vi "shag_start — 9.vi"() -> ()   [LabVIEW 2016]
uses:
  <vilib>/Instr/_visa.llb/VISA Configure Serial Port (Instr).vi
panel:
  out "положение в мин 4":i32
  out "text4":string
  out "4":i32
  out "3":i32
  out "положение в мин 3":i32
  out "text3":string
  out "text":string
  out "2":i32
  out "1":i32
  out "text2":string
  out "положение в мин 2":i32
  out "положение в мин 1":i32
  in  "all":T1(tab)
  out "положение шд 2":i32(knob) scale=-10.0..190.0
  out "текущее положение 2":string
  out "положение в минутах 2":string
  in  "Минуты 2":i32 min=-600 max=11400
  in  "Stop двигатель 2":bool
  in  "Вращение по градусам +  2":bool
  in  "Вращение по градусам -  2":bool
  in  "Вернуться в нулевое положение 2":bool
  in  "Задать текущее положение нулевым 2":bool
  in  "Установка минут 2":bool
  in  "Блокировать трубку №2":bool
  out "положение шд":i32(knob) scale=-10.0..190.0
  out "текущее положение":string
  out "положение в минутах 1":string
  in  "Минуты":i32 min=-600 max=11400
  in  "Stop двигатель":bool
  in  "Вращение по градусам +":bool
  in  "Вращение по градусам -":bool
  in  "Вернуться в нулевое положение":bool
  in  "Задать текущее положение нулевым":bool
  in  "Установка минут":bool
  in  "Блокировать зеркало №1":bool
  in  "stop":bool
  out "положение шд 3":i32(knob) scale=-10.0..190.0
  out "текущее положение 3":string
  out "положение в минутах 3":string
  in  "Минуты 3":i32 min=-600 max=11400
  in  "Stop двигатель 3":bool
  in  "Вращение по градусам +  3":bool
  in  "Вращение по градусам -  3":bool
  in  "Вернуться в нулевое положение 3":bool
  in  "Задать текущее положение нулевым 3":bool
  in  "Установка минут 3":bool
  in  "Блокировать стол №3":bool caption="Блокировать трубку №2"
  out "положение шд 4":i32(knob) scale=-10.0..190.0
  out "текущее положение 4":string
  out "положение в минутах 4":string
  in  "Минуты 4":i32 min=-600 max=11400
  in  "Stop двигатель 4":bool
  in  "Вращение по градусам +  4":bool
  in  "Вращение по градусам -  4":bool
  in  "Вернуться в нулевое положение 4":bool
  in  "Задать текущее положение нулевым 4":bool
  in  "Установка минут 4":bool
  in  "Блокировать стол №3 2":bool caption="Блокировать трубку №2"
  in  "Выберете COM порт":refnum<visa-resource-name>="COM1"
  in  "Скорость обмена данными":u32(ring)=19200 items=["9600"=9600, "19200"=19200, "38400"=38400, "57600"=57600]
  in  "Число бит на символ":u16=8 min=5 max=8 step=1
  in  "Контроль чётности":enum16{"None", "Odd", "Even", "Mark", "Space"}(ring)
  in  "Стоповый бит":u16(ring)=10 items=["1.0"=10, "1.5"=15, "2.0"=20]
  in  "Контроль переполнения":u16(ring) items=["None"=0, "XON/XOFF"=1, "RTS/CTS"=2, "DTR/DSR"=4]
  # "1 - адресс 1 двигателя\n2 - адресс 2 двигателя\n$0MV\\01+   - запуск всех двигателей в положительном направлении \n$0MS\\00   - остановка всех двигателей\n$0MJ\\04+\\00\\00\\01   - 1 шаг всех двигателей\n$0SS\\01\\10   - скорость 10 для всех двигателей"
  # "Ренгеновская трубка №2"
  # "Положение:"
  # "Зеркало №1"
  # "Положение:"
  # "Поворотный стол №3"
  # "Положение:"
  # "Счётчик №4"
  # "Положение:"
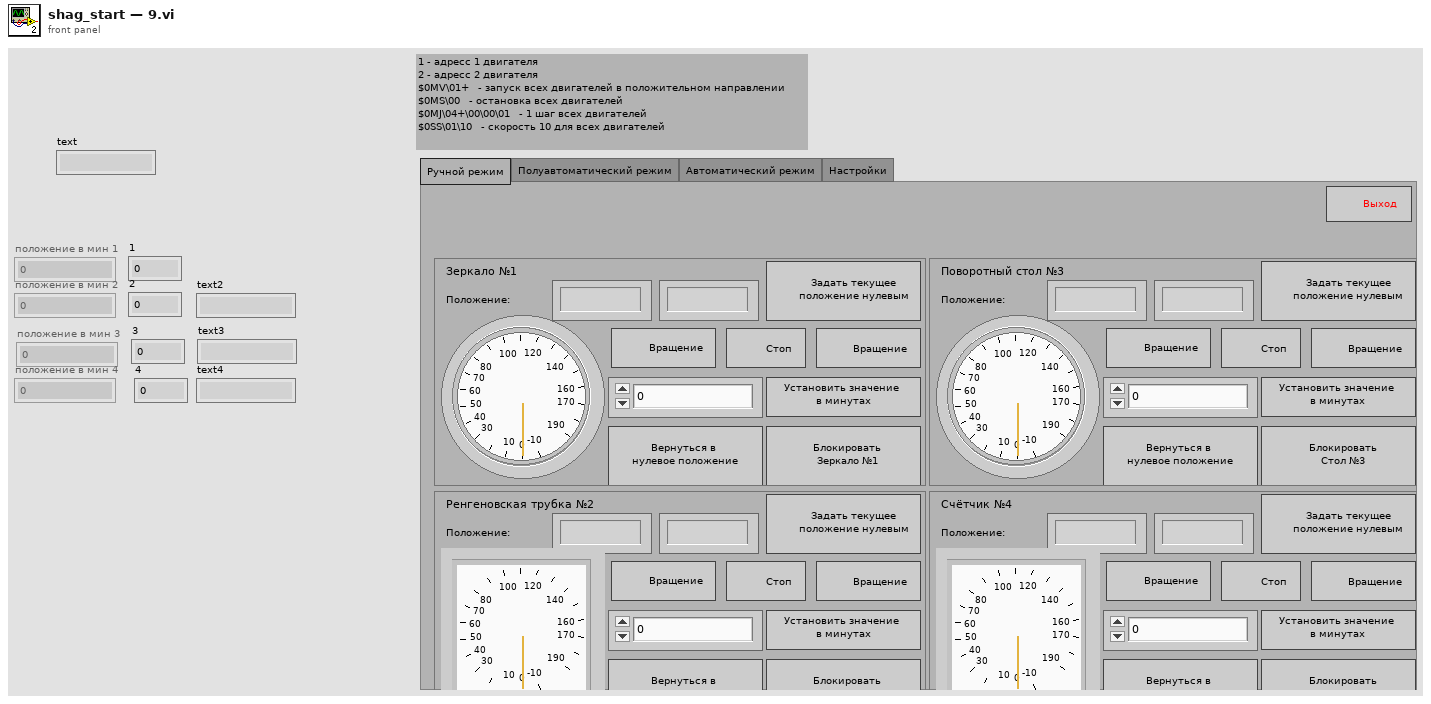
[diagram p1: front panel]
types:
  T1 = enum32{"Ручной режим", "Полуавтоматический режим", "Автоматический режим", "Настройки"}
  T2 = enum16{"open", "replace", "create", "open or create", "replace or create", "replace or create with confirmation"}
  T3 = enum8{"Enabled", "Disabled", "Disabled and Grayed Out"}
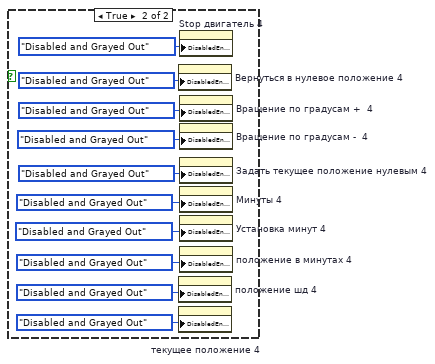
[diagram p2: hidden frame]
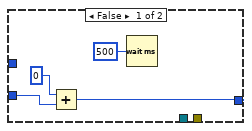
[diagram p4: hidden frame]
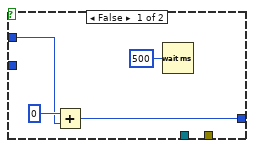
[diagram p5: hidden frame]
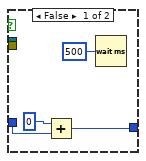
[diagram p7: hidden frame]
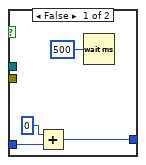
[diagram p8: hidden frame]
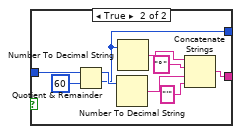
[diagram p9: hidden frame]
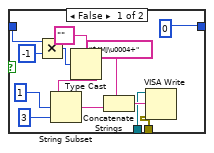
[diagram p11: hidden frame]
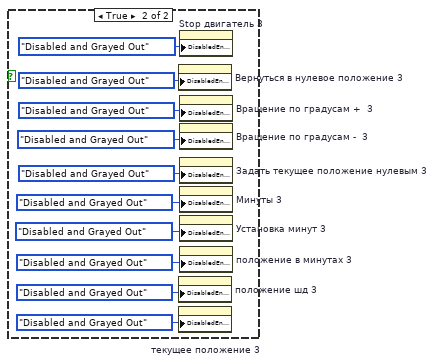
[diagram p13: hidden frame]
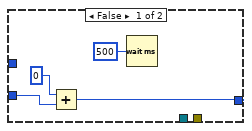
[diagram p15: hidden frame]
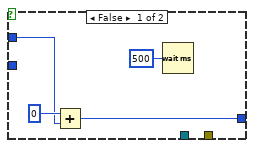
[diagram p16: hidden frame]
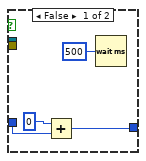
[diagram p18: hidden frame]
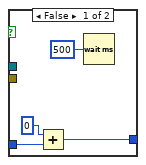
[diagram p19: hidden frame]
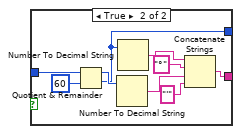
[diagram p20: hidden frame]
diagram:
  n1 = call-poly "VISA Configure Serial Port"("VISA resource name"="Выберете COM порт", "baud rate (9600)"="Скорость обмена данными", "data bits (8)"="Число бит на символ", "parity (0:none)"="Контроль чётности", "stop bits (10: 1 bit)"="Стоповый бит", "flow control (0:none)"="Контроль переполнения") -> ("VISA resource name out"=w32:refnum<visa-resource-name>, "error out"=w31:errorcluster)  [unwired: 8 in]
  n2 = Boolean To (0,1)(Boolean=FALSE ("DTR Write")) -> (0, 1=w33:i16)
  n3 = Boolean To (0,1)(Boolean=FALSE ("DTR Write")) -> (0, 1=w34:i16)
  n4 = property class="Instr"(reference=w32, error in=w31, "Serial Settings:Modem Line Settings:Line DTR State"=w33, "Serial Settings:Modem Line Settings:Line RTS State"=w34) -> (reference out=w30:refnum<visa-resource-name>, error out=w29:errorcluster)
  n5 = flat-sequence {
    tunnel: w30 -> [w63]
    tunnel: w29 -> [w62]
    tunnel: [w63] -> w28
    tunnel: [w62] -> w27
    tunnel: [w58] -> w18
    tunnel: [w66] -> w17
    tunnel: w28 -> [w66]
    tunnel: w27 -> [w65]
    tunnel: [w65] -> w15
    tunnel: [w66] -> w13
    tunnel: [w65] -> w11
    tunnel: w18 -> [w67]
    tunnel: [w65] -> w6
    tunnel: [w66] -> w5
    tunnel: [w66] -> w3
    tunnel: [w65] -> w1
    tunnel: w17 -> [w80]
    tunnel: [w80] -> w16
    tunnel: w15 -> [w79]
    tunnel: [w79] -> w14
    tunnel: w13 -> [w72]
    tunnel: [w72] -> w12
    tunnel: w11 -> [w74]
    tunnel: [w74] -> w10
    tunnel: [w75] -> w9
    tunnel: [w73] -> w8
    tunnel: [w71] -> w7
    tunnel: w6 -> [w73]
    tunnel: w5 -> [w71]
    tunnel: [w70] -> w4
    tunnel: w3 -> [w70]
    tunnel: [w69] -> w2
    tunnel: w1 -> [w69]
    tunnel: w16 -> [w90]
    tunnel: w14 -> [w89]
    tunnel: w12 -> [w85]
    tunnel: w10 -> [w88]
    tunnel: w9 -> [w87]
    tunnel: w8 -> [w84]
    tunnel: w7 -> [w83]
    tunnel: w4 -> [w82]
    tunnel: w2 -> [w81]
    frame #0 {
      n6 = VISA Write(VISA resource name=w63, write buffer="$0SS\u0001\u0010", error in (no error)=w62) -> ()  [unwired: 3 out]
      n7 = Open/Create/Replace File(file path (use dialog)=path "C:/Users/User/Desktop/shagovi_dvigatel/test_text_file", operation (0:open)=T2."open", access (0:read/write)=enum16{"read/write", "read-only", "write-only"}."read-only") -> (refnum out=w57:refnum<file>)  [unwired: 3 in, 2 out]
      n8 = Read from Text File(file (use dialog)=w57) -> (refnum out=w58:refnum<file>, text=w44:string)  [unwired: 3 in, 2 out]
      "text" <- w44
      n9 = Spreadsheet String To Array(delimiter (Tab)=" ", format string="%5f", spreadsheet string=w44) -> (array=w54:dbl[][])  [unwired: 1 in]
      n10 = Index Array(array=w54, index (row)=0 ("index")) -> (element=w52:dbl[])  [unwired: 1 in]
      n11 = Decimate 1D Array(w52) -> (w49:dbl[], w40:dbl[], w39:dbl[], w35:dbl[])
      n12 = Index Array(array=w35, index=0) -> (element=w37:dbl)
      n13 = Index Array(array=w39, index=0) -> (element=w42:dbl)
      n14 = Index Array(array=w40, index=0) -> (element=w48:dbl)
      n15 = To Long Integer(number=w37) -> (32bit integer=→"4":i32)
      n16 = To Long Integer(number=w42) -> (32bit integer=→"3":i32)
      n17 = Index Array(array=w49, index=0) -> (element=w47:dbl)
      n18 = To Long Integer(number=w48) -> (32bit integer=→"2":i32)
      n19 = To Long Integer(number=w47) -> (32bit integer=→"1":i32)
    }
    frame #1 {
      n20 = Close File(refnum=w67) -> ()  [unwired: 1 in, 2 out]
      n21 = Wait (ms)(milliseconds to wait=u32 500) -> ()  [unwired: 1 out]
    }
    frame #2 {
      n22 = Open/Create/Replace File(file path (use dialog)=path "C:/Users/User/Desktop/shagovi_dvigatel/test_text_file", operation (0:open)=T2."replace or create", access (0:read/write)=enum16{"read/write", "read-only", "write-only"}."write-only") -> (refnum out=w75:refnum<file>)  [unwired: 3 in, 2 out]
    }
    frame #3 {
      n23 = while {
        tunnel: w90 -> [w197]
        tunnel: w89 -> [w196]
        shift-right: [w192] -> _
        shift-left: _ -> [w201]
        shift-right: [w193] -> _
        shift-left: _ -> [w200]
        shift-right: [w194] -> _
        shift-left: _ -> [w199]
        shift-right: [w195] -> _
        shift-left: _ -> [w198]
        tunnel: w88 -> [w166]
        shift-right: [w188] -> w86
        shift-left: w87 -> [w189]
        tunnel: w85 -> [w165]
        shift-right: [w161] -> _
        shift-left: _ -> [w162]
        shift-right: [w159] -> _
        shift-left: _ -> [w160]
        shift-right: [w157] -> _
        shift-left: _ -> [w158]
        shift-right: [w155] -> _
        shift-left: _ -> [w156]
        tunnel: w84 -> [w133]
        tunnel: w83 -> [w132]
        shift-right: [w129] -> _
        shift-left: _ -> [w130]
        shift-right: [w127] -> _
        shift-left: _ -> [w128]
        shift-right: [w125] -> _
        shift-left: _ -> [w126]
        shift-right: [w123] -> _
        shift-left: _ -> [w124]
        tunnel: w82 -> [w101]
        tunnel: w81 -> [w100]
        shift-right: [w97] -> _
        shift-left: _ -> [w98]
        shift-right: [w95] -> _
        shift-left: _ -> [w96]
        shift-right: [w93] -> _
        shift-left: _ -> [w94]
        shift-right: [w91] -> _
        shift-left: _ -> [w92]
        stop <- "stop" stop-if-true
        # "Управление вращением"
        # "Управление вращением"
        n24 = flat-sequence {
          tunnel: w133 -> [w520]
          tunnel: w132 -> [w521]
          tunnel: [w521] -> w154
          tunnel: [w520] -> w153
          tunnel: ["Вращение по градусам +  3"] -> w152
          tunnel: ["Вращение по градусам -  3"] -> w151
          tunnel: ["Вернуться в нулевое положение 3"] -> w150
          tunnel: ["Задать текущее положение нулевым 3"] -> w149
          tunnel: ["Установка минут 3"] -> w148
          tunnel: w154 -> [w545]
          tunnel: w153 -> [w529]
          tunnel: [w568] -> w147
          tunnel: w130 -> [w565]
          tunnel: w128 -> [w567]
          tunnel: [w566] -> w146
          tunnel: w126 -> [w564]
          tunnel: w124 -> [w563]
          tunnel: w152 -> [w549]
          tunnel: w151 -> [w548]
          tunnel: [w562] -> w145
          tunnel: [w561] -> w144
          tunnel: [w546] -> w143
          tunnel: w150 -> [w546]
          tunnel: [w529] -> w142
          tunnel: [w545] -> w141
          tunnel: [w544] -> w140
          tunnel: w149 -> [w544]
          tunnel: w148 -> [w538]
          tunnel: [w527] -> w139
          tunnel: w147 -> [w652]
          tunnel: w146 -> [w653]
          tunnel: [w670] -> w138
          tunnel: [w668] -> w137
          tunnel: w145 -> [w654]
          tunnel: w144 -> [w655]
          tunnel: [w659] -> w136
          tunnel: [w666] -> w135
          tunnel: w143 -> [w662]
          tunnel: w142 -> [w658]
          tunnel: w141 -> [w657]
          tunnel: w140 -> [w656]
          tunnel: [w656] -> w134
          tunnel: w139 -> [w642]
          tunnel: [w749] -> w129
          tunnel: [w746] -> w127
          tunnel: w138 -> [w748]
          tunnel: w137 -> [w747]
          tunnel: [w745] -> w125
          tunnel: [w744] -> w123
          tunnel: w136 -> [w743]
          tunnel: w135 -> [w742]
          tunnel: w134 -> [w741]
          frame #0 {
            n25 = Wait Until Next ms Multiple(millisecond multiple=u32 300) -> ()  [unwired: 1 out]
          }
          frame #1 {
            # "Остановка двигателя"
            n26 = Greater?(x="Минуты 3", y=0) -> (0:w536:bool)
            n27 = case shown="True" "Stop двигатель 3" {
              tunnel: w545 -> [_ w616]
              tunnel: w529 -> [_ w615]
              frame False {
              }
              frame True {
                n28 = Wait (ms)(milliseconds to wait=u32 500) -> ()  [unwired: 1 out]
                n29 = VISA Write(VISA resource name=w616, write buffer="$3MS\u0001", error in (no error)=w615) -> ()  [unwired: 3 out]
              }
            }
            n30 = Not Equal?(x="Минуты 3", y=0) -> (x != y?=w535:bool)
            n31 = local read "положение в мин 3"() -> (w528:i32)
            n32 = Add(x="Минуты 3", y=w528) -> (x+y=w559:i32)
            n33 = Add(x="Минуты 3", y=w528) -> (x+y=w531:i32)
            n34 = Not Equal?(x="Минуты 3", y=0) -> (x != y?=w533:bool)
            n35 = Add(x=w528, y=60) -> (x+y=w554:i32)
            n36 = Subtract(x=w528, y=60) -> (x-y=w541:i32)
            n37 = Not(x=w536) -> (.not. x?=w537:bool)
            n38 = Greater Or Equal?(x=w531, y=-600) -> (x >= y?=w532:bool)
            n39 = Less Or Equal?(x=w559, y=11400) -> (x <= y?=w534:bool)
            n40 = Less Or Equal?(x=w554, y=11390) -> (x <= y?=w551:bool)
            n41 = Greater Or Equal?(x=w541, y=-590) -> (x >= y?=w542:bool)
            n42 = Compound Arithmetic op=AND(w537, w533, w532) -> (w555:bool)
            n43 = And(x=w549, y=w551) -> (x .and. y?=w550:bool)
            n44 = And(x=w548, y=w542) -> (x .and. y?=w547:bool)
            n45 = Compound Arithmetic op=AND(w536, w535, w534) -> (w557:bool)
            n46 = case shown="True" w538 {
              tunnel: [w571 w580] -> w568
              tunnel: w567 -> [w570 w579]
              tunnel: [w570 w578] -> w566
              tunnel: w565 -> [w571 w577]
              tunnel: w557 -> [_ w576]
              tunnel: w555 -> [_ w575]
              tunnel: w529 -> [_ w574]
              tunnel: w545 -> [_ w573]
              tunnel: "Минуты 3" -> [_ w572]
              frame False {
              }
              frame True {
                n47 = case shown="True" w576 {
                  tunnel: [w601 w607] -> w580
                  tunnel: w577 -> [w600 w606]
                  tunnel: w574 -> [_ w605]
                  tunnel: w573 -> [_ w604]
                  tunnel: w572 -> [_ w603]
                  frame False {
                    n48 = Add(x=0, y=w600) -> (x+y=w601:i32)
                    n49 = Wait (ms)(milliseconds to wait=u32 500) -> ()  [unwired: 1 out]
                  }
                  frame True {
                    n50 = Type Cast(type="", x=w603) -> (*(type *) &x=w610:string)
                    n51 = Add(x=w603, y=w606) -> (x+y=w607:i32)
                    n52 = String Subset(string=w610, offset (0)=1, length (rest)=3 ("length (rest)")) -> (substring=w609:string)
                    n53 = Concatenate Strings("$3MJ\u0004+" ("write buffer"), w609) -> (w613:string)
                    n54 = VISA Write(VISA resource name=w604, write buffer=w613, error in (no error)=w605) -> ()  [unwired: 3 out]
                  }
                }
                n55 = case shown="True" w575 {
                  tunnel: [w583 w589] -> w578
                  tunnel: w579 -> [w582 w588]
                  tunnel: w573 -> [_ w591]
                  tunnel: w574 -> [_ w590]
                  tunnel: w572 -> [_ w585]
                  frame False {
                    n56 = Add(x=0, y=w582) -> (x+y=w583:i32)
                    n57 = Wait (ms)(milliseconds to wait=u32 500) -> ()  [unwired: 1 out]
                  }
                  frame True {
                    n58 = Multiply(x=w585, y=-1) -> (x*y=w587:i32)
                    n59 = Type Cast(type="", x=w587) -> (*(type *) &x=w594:string)
                    n60 = Add(x=w588, y=w585) -> (x+y=w589:i32)
                    n61 = String Subset(string=w594, offset (0)=1, length (rest)=3 ("length (rest)")) -> (substring=w593:string)
                    n62 = Concatenate Strings("$3MJ\u0004-" ("write buffer"), w593) -> (w597:string)
                    n63 = VISA Write(VISA resource name=w591, write buffer=w597, error in (no error)=w590) -> ()  [unwired: 3 out]
                  }
                }
              }
            }
            n64 = case shown="True" w550 {
              tunnel: [w631 w638] -> w562
              tunnel: w564 -> [w630 w633]
              tunnel: w545 -> [_ w634]
              tunnel: w529 -> [_ w635]
              frame False {
                n65 = Add(x=0, y=w630) -> (x+y=w631:i32)
                n66 = Wait (ms)(milliseconds to wait=u32 500) -> ()  [unwired: 1 out]
              }
              frame True {
                n67 = VISA Write(VISA resource name=w634, write buffer="$3MJ\u0004+\u0000\u0000<", error in (no error)=w635) -> ()  [unwired: 3 out]
                n68 = Add(x=60, y=w633) -> (x+y=w638:i32)
              }
            }
            n69 = case shown="True" w547 {
              tunnel: [w621 w624] -> w561
              tunnel: w563 -> [w620 w623]
              tunnel: w545 -> [_ w627]
              tunnel: w529 -> [_ w626]
              frame False {
                n70 = Add(x=0, y=w620) -> (x+y=w621:i32)
                n71 = Wait (ms)(milliseconds to wait=u32 500) -> ()  [unwired: 1 out]
              }
              frame True {
                n72 = Subtract(x=w623, y=60 ("x")) -> (x-y=w624:i32)
                n73 = VISA Write(VISA resource name=w627, write buffer="$3MJ\u0004-\u0000\u0000<", error in (no error)=w626) -> ()  [unwired: 3 out]
              }
            }
            n74 = for {
              N: 1 -> [_]
              tunnel: [w569] -> w525 mode=indexing
              n75 = local read "3"() -> (w569:i32)
            }
            n76 = Index Array(array=w525, index=0) -> (element=w527:i32)
          }
          frame #2 {
            # "Нулевое положение"
            n77 = Add(x=w654, y=w655) -> (x+y=w663:i32)
            n78 = Add(x=w652, y=w653) -> (x+y=w667:i32)
            n79 = Add(x=w667, y=w663) -> (x+y=w648:i32)
            n80 = Add(x=w648, y=w642) -> (x+y=w647:i32)
            n81 = Not Equal?(x=w647, y=0 ("x")) -> (x != y?=w660:bool)
            n82 = And(x=w660, y=w662) -> (x .and. y?=w669:bool)
            n83 = case shown="True" w669 {
              tunnel: [w694 w716] -> w644
              tunnel: w652 -> [w698 w713]
              tunnel: [w698 w712] -> w670
              tunnel: [w697 w711] -> w668
              tunnel: w647 -> [w694 w705]
              tunnel: [w695 w707] -> w666
              tunnel: [w696 w704] -> w659
              tunnel: w653 -> [w697 w703]
              tunnel: w658 -> [_ w702]
              tunnel: w657 -> [_ w701]
              tunnel: w654 -> [w696 w700]
              tunnel: w655 -> [w695 w699]
              frame False {
              }
              frame True {
                n84 = Greater?(x=w705, y=0) -> (0:w706:bool)
                n85 = Multiply(x=w699, y=0) -> (x*y=w707:i32)
                n86 = Multiply(x=w703, y=0) -> (x*y=w711:i32)
                n87 = case shown="False" w706 {
                  tunnel: w705 -> [w721 w734]
                  tunnel: [0 0] -> w716
                  tunnel: w701 -> [w718 w731]
                  tunnel: w702 -> [w717 w730]
                  frame False {
                    n88 = Multiply(x=w721, y=-1) -> (x*y=w719:i32)
                    n89 = Type Cast(type="", x=w719) -> (*(type *) &x=w725:string)
                    n90 = String Subset(string=w725, offset (0)=1, length (rest)=3 ("length (rest)")) -> (substring=w724:string)
                    n91 = Concatenate Strings("$3MJ\u0004+" ("write buffer"), w724) -> (w728:string)
                    n92 = VISA Write(VISA resource name=w718, write buffer=w728, error in (no error)=w717) -> ()  [unwired: 3 out]
                  }
                  frame True {
                    n93 = Type Cast(type="", x=w734) -> (*(type *) &x=w737:string)
                    n94 = String Subset(string=w737, offset (0)=1, length (rest)=3 ("length (rest)")) -> (substring=w736:string)
                    n95 = Concatenate Strings("$3MJ\u0004-" ("write buffer"), w736) -> (w732:string)
                    n96 = VISA Write(VISA resource name=w731, write buffer=w732, error in (no error)=w730) -> ()  [unwired: 3 out]
                  }
                }
                n97 = Multiply(x=w700, y=0) -> (x*y=w704:i32)
                n98 = Multiply(x=w713, y=0) -> (x*y=w712:i32)
              }
            }
            "положение в мин 3" <- w644
            n99 = Greater?(x=w644, y=0) -> (0:w665:bool)
            n100 = Number To Decimal String(number=w644, width (-)=i16 1) -> (decimal integer string=w650:string)
            n101 = case shown="False" w665 {
              tunnel: w644 -> [w677 w693]
              tunnel: [w681 w687] -> w641
              tunnel: [w671 w685] -> w639
              frame False {
                n102 = Multiply(x=-1, y=w677) -> (x*y=w676:i32)
                n103 = Quotient & Remainder(x=w676, y=60) -> (x-y*floor(x/y)=w680:i32, floor(x/y)=w672:i32)
                n104 = Multiply(x=-1, y=w672) -> (x*y=w671:i32)
                n105 = Number To Decimal String(number=w672) -> (decimal integer string=w678:string)  [unwired: 1 in]
                n106 = Number To Decimal String(number=w680) -> (decimal integer string=w679:string)  [unwired: 1 in]
                n107 = Concatenate Strings("-" ("string"), w678, "°" ("string"), w679, "'" ("string")) -> (w681:string)
              }
              frame True {
                n108 = Quotient & Remainder(x=w693, y=60) -> (x-y*floor(x/y)=w686:i32, floor(x/y)=w685:i32)
                n109 = Number To Decimal String(number=w686) -> (decimal integer string=w688:string)  [unwired: 1 in]
                n110 = Number To Decimal String(number=w685) -> (decimal integer string=w689:string)  [unwired: 1 in]
                n111 = Concatenate Strings(w689, "°" ("string"), w688, "'" ("string")) -> (w687:string)
              }
            }
            "текущее положение 3" <- w641
            "положение шд 3" <- w639
            n112 = Concatenate Strings(w650, "'" ("string")) -> (→"положение в минутах 3":string)
            n113 = Format Into String(w644) -> (resulting string=w645:string)  [unwired: 3 in, 1 out]
            n114 = call <vilib>:"Space Constant.vi"() -> ("String"=w643:string)
            n115 = Concatenate Strings(w643, w645) -> (→"text3":string)
          }
          frame #3 {
            # "Задача нуля"
            n116 = case shown="True" w741 {
              tunnel: [w753 w764] -> w749
              tunnel: w748 -> [w753 w765]
              tunnel: w747 -> [w752 w761]
              tunnel: [w752 w760] -> w746
              tunnel: [w751 w757] -> w745
              tunnel: [w750 w756] -> w744
              tunnel: w743 -> [w751 w755]
              tunnel: w742 -> [w750 w754]
              frame False {
              }
              frame True {
                n117 = Multiply(x=w761, y=0) -> (x*y=w760:i32)
                n118 = Multiply(x=w765, y=0) -> (x*y=w764:i32)
                n119 = Multiply(x=w754, y=0) -> (x*y=w756:i32)
                n120 = Multiply(x=w755, y=0) -> (x*y=w757:i32)
              }
            }
          }
        }
        n121 = flat-sequence {
          tunnel: w196 -> [w1064]
          tunnel: w197 -> [w1065]
          tunnel: [w1065] -> w221
          tunnel: [w1064] -> w220
          tunnel: ["Вращение по градусам +"] -> w219
          tunnel: ["Вращение по градусам -"] -> w218
          tunnel: ["Вернуться в нулевое положение"] -> w217
          tunnel: ["Задать текущее положение нулевым"] -> w216
          tunnel: ["Установка минут"] -> w215
          tunnel: w221 -> [w1089]
          tunnel: w220 -> [w1071]
          tunnel: [w1112] -> w214
          tunnel: w201 -> [w1109]
          tunnel: w200 -> [w1111]
          tunnel: [w1110] -> w213
          tunnel: w199 -> [w1108]
          tunnel: w198 -> [w1107]
          tunnel: w219 -> [w1093]
          tunnel: w218 -> [w1092]
          tunnel: [w1106] -> w212
          tunnel: [w1105] -> w211
          tunnel: [w1090] -> w210
          tunnel: w217 -> [w1090]
          tunnel: [w1071] -> w209
          tunnel: [w1089] -> w208
          tunnel: [w1088] -> w207
          tunnel: w216 -> [w1088]
          tunnel: w215 -> [w1082]
          tunnel: [w1069] -> w190
          tunnel: w214 -> [w1194]
          tunnel: w213 -> [w1195]
          tunnel: [w1214] -> w206
          tunnel: [w1212] -> w205
          tunnel: w212 -> [w1196]
          tunnel: w211 -> [w1197]
          tunnel: [w1203] -> w204
          tunnel: [w1210] -> w203
          tunnel: w210 -> [w1206]
          tunnel: w209 -> [w1202]
          tunnel: w208 -> [w1201]
          tunnel: w207 -> [w1199]
          tunnel: [w1199] -> w202
          tunnel: [w1188] -> _
          tunnel: "stop" -> [w1191]
          tunnel: w189 -> [w1188]
          tunnel: w190 -> [w1183]
          tunnel: [w1184] -> w188
          tunnel: [w1302] -> w192
          tunnel: [w1299] -> w193
          tunnel: w206 -> [w1301]
          tunnel: w205 -> [w1300]
          tunnel: [w1298] -> w194
          tunnel: [w1297] -> w195
          tunnel: w204 -> [w1296]
          tunnel: w203 -> [w1295]
          tunnel: w202 -> [w1294]
          frame #0 {
            n122 = Wait Until Next ms Multiple(millisecond multiple=u32 300) -> ()  [unwired: 1 out]
          }
          frame #1 {
            # "Остановка двигателя"
            n123 = Greater?(x="Минуты", y=0) -> (0:w1080:bool)
            n124 = case shown="True" "Stop двигатель" {
              tunnel: w1089 -> [_ w1160]
              tunnel: w1071 -> [_ w1159]
              frame False {
              }
              frame True {
                n125 = Wait (ms)(milliseconds to wait=u32 500) -> ()  [unwired: 1 out]
                n126 = VISA Write(VISA resource name=w1160, write buffer="$1MS\u0001", error in (no error)=w1159) -> ()  [unwired: 3 out]
              }
            }
            n127 = Not Equal?(x="Минуты", y=0) -> (x != y?=w1079:bool)
            n128 = local read "положение в мин 1"() -> (w1070:i32)
            n129 = Add(x="Минуты", y=w1070) -> (x+y=w1103:i32)
            n130 = Add(x="Минуты", y=w1070) -> (x+y=w1074:i32)
            n131 = Not Equal?(x="Минуты", y=0) -> (x != y?=w1077:bool)
            n132 = Add(x=w1070, y=60) -> (x+y=w1098:i32)
            n133 = Subtract(x=w1070, y=60) -> (x-y=w1085:i32)
            n134 = Not(x=w1080) -> (.not. x?=w1081:bool)
            n135 = Greater Or Equal?(x=w1074, y=-600) -> (x >= y?=w1075:bool)
            n136 = Less Or Equal?(x=w1103, y=11400) -> (x <= y?=w1078:bool)
            n137 = Less Or Equal?(x=w1098, y=11390) -> (x <= y?=w1095:bool)
            n138 = Greater Or Equal?(x=w1085, y=-590) -> (x >= y?=w1086:bool)
            n139 = Compound Arithmetic op=AND(w1081, w1077, w1075) -> (w1099:bool)
            n140 = And(x=w1093, y=w1095) -> (x .and. y?=w1094:bool)
            n141 = And(x=w1092, y=w1086) -> (x .and. y?=w1091:bool)
            n142 = Compound Arithmetic op=AND(w1080, w1079, w1078) -> (w1101:bool)
            n143 = case shown="True" w1082 {
              tunnel: [w1115 w1124] -> w1112
              tunnel: w1111 -> [w1114 w1123]
              tunnel: [w1114 w1122] -> w1110
              tunnel: w1109 -> [w1115 w1121]
              tunnel: w1101 -> [_ w1120]
              tunnel: w1099 -> [_ w1119]
              tunnel: w1071 -> [_ w1118]
              tunnel: w1089 -> [_ w1117]
              tunnel: "Минуты" -> [_ w1116]
              frame False {
              }
              frame True {
                n144 = case shown="True" w1120 {
                  tunnel: [w1145 w1151] -> w1124
                  tunnel: w1121 -> [w1144 w1150]
                  tunnel: w1118 -> [_ w1149]
                  tunnel: w1117 -> [_ w1148]
                  tunnel: w1116 -> [_ w1147]
                  frame False {
                    n145 = Add(x=0, y=w1144) -> (x+y=w1145:i32)
                    n146 = Wait (ms)(milliseconds to wait=u32 500) -> ()  [unwired: 1 out]
                  }
                  frame True {
                    n147 = Type Cast(type="", x=w1147) -> (*(type *) &x=w1154:string)
                    n148 = Add(x=w1147, y=w1150) -> (x+y=w1151:i32)
                    n149 = String Subset(string=w1154, offset (0)=1, length (rest)=3 ("length (rest)")) -> (substring=w1153:string)
                    n150 = Concatenate Strings("$1MJ\u0004+" ("write buffer"), w1153) -> (w1157:string)
                    n151 = VISA Write(VISA resource name=w1148, write buffer=w1157, error in (no error)=w1149) -> ()  [unwired: 3 out]
                  }
                }
                n152 = case shown="True" w1119 {
                  tunnel: [w1127 w1133] -> w1122
                  tunnel: w1123 -> [w1126 w1132]
                  tunnel: w1117 -> [_ w1135]
                  tunnel: w1118 -> [_ w1134]
                  tunnel: w1116 -> [_ w1129]
                  frame False {
                    n153 = Add(x=0, y=w1126) -> (x+y=w1127:i32)
                    n154 = Wait (ms)(milliseconds to wait=u32 500) -> ()  [unwired: 1 out]
                  }
                  frame True {
                    n155 = Multiply(x=w1129, y=-1) -> (x*y=w1131:i32)
                    n156 = Type Cast(type="", x=w1131) -> (*(type *) &x=w1138:string)
                    n157 = Add(x=w1132, y=w1129) -> (x+y=w1133:i32)
                    n158 = String Subset(string=w1138, offset (0)=1, length (rest)=3 ("length (rest)")) -> (substring=w1137:string)
                    n159 = Concatenate Strings("$1MJ\u0004-" ("write buffer"), w1137) -> (w1141:string)
                    n160 = VISA Write(VISA resource name=w1135, write buffer=w1141, error in (no error)=w1134) -> ()  [unwired: 3 out]
                  }
                }
              }
            }
            n161 = case shown="True" w1094 {
              tunnel: [w1175 w1182] -> w1106
              tunnel: w1108 -> [w1174 w1177]
              tunnel: w1089 -> [_ w1178]
              tunnel: w1071 -> [_ w1179]
              frame False {
                n162 = Add(x=0, y=w1174) -> (x+y=w1175:i32)
                n163 = Wait (ms)(milliseconds to wait=u32 500) -> ()  [unwired: 1 out]
              }
              frame True {
                n164 = VISA Write(VISA resource name=w1178, write buffer="$1MJ\u0004+\u0000\u0000<", error in (no error)=w1179) -> ()  [unwired: 3 out]
                n165 = Add(x=60, y=w1177) -> (x+y=w1182:i32)
              }
            }
            n166 = case shown="True" w1091 {
              tunnel: [w1165 w1168] -> w1105
              tunnel: w1107 -> [w1164 w1167]
              tunnel: w1089 -> [_ w1171]
              tunnel: w1071 -> [_ w1170]
              frame False {
                n167 = Add(x=0, y=w1164) -> (x+y=w1165:i32)
                n168 = Wait (ms)(milliseconds to wait=u32 500) -> ()  [unwired: 1 out]
              }
              frame True {
                n169 = Subtract(x=w1167, y=60 ("x")) -> (x-y=w1168:i32)
                n170 = VISA Write(VISA resource name=w1171, write buffer="$1MJ\u0004-\u0000\u0000<", error in (no error)=w1170) -> ()  [unwired: 3 out]
              }
            }
            n171 = for {
              N: 1 -> [_]
              tunnel: [w1113] -> w1067 mode=indexing
              n172 = local read "1"() -> (w1113:i32)
            }
            n173 = Index Array(array=w1067, index=0) -> (element=w1069:i32)
          }
          frame #2 {
            # "Нулевое положение"
            n174 = Add(x=w1196, y=w1197) -> (x+y=w1207:i32)
            n175 = Add(x=w1194, y=w1195) -> (x+y=w1211:i32)
            n176 = Add(x=w1211, y=w1207) -> (x+y=w1186:i32)
            n177 = Add(x=w1186, y=w1183) -> (x+y=w1185:i32)
            n178 = Not Equal?(x=w1185, y=0 ("x")) -> (x != y?=w1204:bool)
            n179 = And(x=w1204, y=w1206) -> (x .and. y?=w1213:bool)
            n180 = case shown="True" w1213 {
              tunnel: [w1247 w1269] -> w1187
              tunnel: w1194 -> [w1251 w1266]
              tunnel: [w1251 w1265] -> w1214
              tunnel: [w1250 w1264] -> w1212
              tunnel: w1185 -> [w1247 w1258]
              tunnel: [w1248 w1260] -> w1210
              tunnel: [w1249 w1257] -> w1203
              tunnel: w1195 -> [w1250 w1256]
              tunnel: w1202 -> [_ w1255]
              tunnel: w1201 -> [_ w1254]
              tunnel: w1196 -> [w1249 w1253]
              tunnel: w1197 -> [w1248 w1252]
              frame False {
              }
              frame True {
                n181 = Greater?(x=w1258, y=0) -> (0:w1259:bool)
                n182 = Multiply(x=w1252, y=0) -> (x*y=w1260:i32)
                n183 = Multiply(x=w1256, y=0) -> (x*y=w1264:i32)
                n184 = case shown="True" w1259 {
                  tunnel: w1258 -> [w1274 w1287]
                  tunnel: [0 0] -> w1269
                  tunnel: w1254 -> [w1271 w1284]
                  tunnel: w1255 -> [w1270 w1283]
                  frame False {
                    n185 = Multiply(x=w1274, y=-1) -> (x*y=w1272:i32)
                    n186 = Type Cast(type="", x=w1272) -> (*(type *) &x=w1278:string)
                    n187 = String Subset(string=w1278, offset (0)=1, length (rest)=3 ("length (rest)")) -> (substring=w1277:string)
                    n188 = Concatenate Strings("$1MJ\u0004+" ("write buffer"), w1277) -> (w1281:string)
                    n189 = VISA Write(VISA resource name=w1271, write buffer=w1281, error in (no error)=w1270) -> ()  [unwired: 3 out]
                  }
                  frame True {
                    n190 = Type Cast(type="", x=w1287) -> (*(type *) &x=w1290:string)
                    n191 = String Subset(string=w1290, offset (0)=1, length (rest)=3 ("length (rest)")) -> (substring=w1289:string)
                    n192 = Concatenate Strings("$1MJ\u0004-" ("write buffer"), w1289) -> (w1285:string)
                    n193 = VISA Write(VISA resource name=w1284, write buffer=w1285, error in (no error)=w1283) -> ()  [unwired: 3 out]
                  }
                }
                n194 = Multiply(x=w1253, y=0) -> (x*y=w1257:i32)
                n195 = Multiply(x=w1266, y=0) -> (x*y=w1265:i32)
              }
            }
            "положение в мин 1" <- w1187
            n196 = Greater?(x=w1187, y=0) -> (0:w1209:bool)
            n197 = Number To Decimal String(number=w1187, width (-)=i16 1) -> (decimal integer string=w1190:string)
            n198 = case shown="True" w1191 {
              tunnel: w1188 -> [w1215 w1222]
              tunnel: w1187 -> [_ w1223]
              tunnel: [w1215 w1221] -> w1184
              frame False {
              }
              frame True {
                n199 = Format Into String(w1223) -> (resulting string=w1219:string)  [unwired: 3 in, 1 out]
                n200 = local read "text2"() -> (w1218:string)
                n201 = local read "text3"() -> (w1217:string)
                n202 = local read "text4"() -> (w1216:string)
                n203 = Concatenate Strings(w1219, w1218, w1217, w1216) -> (w1220:string)
                n204 = Write to Text File(file (use dialog)=w1222, text=w1220) -> (refnum out=w1221:refnum<file>)  [unwired: 2 in, 2 out]
              }
            }
            n205 = case shown="False" w1209 {
              tunnel: w1187 -> [w1230 w1246]
              tunnel: [w1234 w1240] -> w1200
              tunnel: [w1224 w1238] -> w1198
              frame False {
                n206 = Multiply(x=-1, y=w1230) -> (x*y=w1229:i32)
                n207 = Quotient & Remainder(x=w1229, y=60) -> (x-y*floor(x/y)=w1233:i32, floor(x/y)=w1225:i32)
                n208 = Multiply(x=-1, y=w1225) -> (x*y=w1224:i32)
                n209 = Number To Decimal String(number=w1225) -> (decimal integer string=w1231:string)  [unwired: 1 in]
                n210 = Number To Decimal String(number=w1233) -> (decimal integer string=w1232:string)  [unwired: 1 in]
                n211 = Concatenate Strings("-" ("string"), w1231, "°" ("string"), w1232, "'" ("string")) -> (w1234:string)
              }
              frame True {
                n212 = Quotient & Remainder(x=w1246, y=60) -> (x-y*floor(x/y)=w1239:i32, floor(x/y)=w1238:i32)
                n213 = Number To Decimal String(number=w1239) -> (decimal integer string=w1241:string)  [unwired: 1 in]
                n214 = Number To Decimal String(number=w1238) -> (decimal integer string=w1242:string)  [unwired: 1 in]
                n215 = Concatenate Strings(w1242, "°" ("string"), w1241, "'" ("string")) -> (w1240:string)
              }
            }
            "положение шд" <- w1198
            "текущее положение" <- w1200
            n216 = Concatenate Strings(w1190, "'" ("string")) -> (→"положение в минутах 1":string)
          }
          frame #3 {
            # "Задача нуля"
            n217 = case shown="True" w1294 {
              tunnel: [w1306 w1317] -> w1302
              tunnel: w1301 -> [w1306 w1318]
              tunnel: w1300 -> [w1305 w1314]
              tunnel: [w1305 w1313] -> w1299
              tunnel: [w1304 w1310] -> w1298
              tunnel: [w1303 w1309] -> w1297
              tunnel: w1296 -> [w1304 w1308]
              tunnel: w1295 -> [w1303 w1307]
              frame False {
              }
              frame True {
                n218 = Multiply(x=w1314, y=0) -> (x*y=w1313:i32)
                n219 = Multiply(x=w1318, y=0) -> (x*y=w1317:i32)
                n220 = Multiply(x=w1307, y=0) -> (x*y=w1309:i32)
                n221 = Multiply(x=w1308, y=0) -> (x*y=w1310:i32)
              }
            }
          }
        }
        n222 = flat-sequence {
          tunnel: w166 -> [w792]
          tunnel: w165 -> [w793]
          tunnel: [w793] -> w187
          tunnel: [w792] -> w186
          tunnel: ["Вращение по градусам +  2"] -> w185
          tunnel: ["Вращение по градусам -  2"] -> w184
          tunnel: ["Вернуться в нулевое положение 2"] -> w183
          tunnel: ["Задать текущее положение нулевым 2"] -> w182
          tunnel: ["Установка минут 2"] -> w181
          tunnel: w187 -> [w817]
          tunnel: w186 -> [w801]
          tunnel: [w840] -> w180
          tunnel: w162 -> [w837]
          tunnel: w160 -> [w839]
          tunnel: [w838] -> w179
          tunnel: w158 -> [w836]
          tunnel: w156 -> [w835]
          tunnel: w185 -> [w821]
          tunnel: w184 -> [w820]
          tunnel: [w834] -> w178
          tunnel: [w833] -> w177
          tunnel: [w818] -> w176
          tunnel: w183 -> [w818]
          tunnel: [w801] -> w175
          tunnel: [w817] -> w174
          tunnel: [w816] -> w173
          tunnel: w182 -> [w816]
          tunnel: w181 -> [w810]
          tunnel: [w799] -> w172
          tunnel: w180 -> [w924]
          tunnel: w179 -> [w925]
          tunnel: [w942] -> w171
          tunnel: [w940] -> w170
          tunnel: w178 -> [w926]
          tunnel: w177 -> [w927]
          tunnel: [w931] -> w169
          tunnel: [w938] -> w168
          tunnel: w176 -> [w934]
          tunnel: w175 -> [w930]
          tunnel: w174 -> [w929]
          tunnel: w173 -> [w928]
          tunnel: [w928] -> w167
          tunnel: w172 -> [w911]
          tunnel: [w1021] -> w161
          tunnel: [w1018] -> w159
          tunnel: w171 -> [w1020]
          tunnel: w170 -> [w1019]
          tunnel: [w1017] -> w157
          tunnel: [w1016] -> w155
          tunnel: w169 -> [w1015]
          tunnel: w168 -> [w1014]
          tunnel: w167 -> [w1013]
          frame #0 {
            n223 = Wait Until Next ms Multiple(millisecond multiple=u32 300) -> ()  [unwired: 1 out]
          }
          frame #1 {
            # "Остановка двигателя"
            n224 = Greater?(x="Минуты 2", y=0) -> (0:w808:bool)
            n225 = case shown="True" "Stop двигатель 2" {
              tunnel: w817 -> [_ w888]
              tunnel: w801 -> [_ w887]
              frame False {
              }
              frame True {
                n226 = Wait (ms)(milliseconds to wait=u32 500) -> ()  [unwired: 1 out]
                n227 = VISA Write(VISA resource name=w888, write buffer="$2MS\u0001", error in (no error)=w887) -> ()  [unwired: 3 out]
              }
            }
            n228 = Not Equal?(x="Минуты 2", y=0) -> (x != y?=w807:bool)
            n229 = local read "положение в мин 2"() -> (w800:i32)
            n230 = Add(x="Минуты 2", y=w800) -> (x+y=w831:i32)
            n231 = Add(x="Минуты 2", y=w800) -> (x+y=w803:i32)
            n232 = Not Equal?(x="Минуты 2", y=0) -> (x != y?=w805:bool)
            n233 = Add(x=w800, y=60) -> (x+y=w826:i32)
            n234 = Subtract(x=w800, y=60) -> (x-y=w813:i32)
            n235 = Not(x=w808) -> (.not. x?=w809:bool)
            n236 = Greater Or Equal?(x=w803, y=-600) -> (x >= y?=w804:bool)
            n237 = Less Or Equal?(x=w831, y=11400) -> (x <= y?=w806:bool)
            n238 = Less Or Equal?(x=w826, y=11390) -> (x <= y?=w823:bool)
            n239 = Greater Or Equal?(x=w813, y=-590) -> (x >= y?=w814:bool)
            n240 = Compound Arithmetic op=AND(w809, w805, w804) -> (w827:bool)
            n241 = And(x=w821, y=w823) -> (x .and. y?=w822:bool)
            n242 = And(x=w820, y=w814) -> (x .and. y?=w819:bool)
            n243 = Compound Arithmetic op=AND(w808, w807, w806) -> (w829:bool)
            n244 = case shown="True" w810 {
              tunnel: [w843 w852] -> w840
              tunnel: w839 -> [w842 w851]
              tunnel: [w842 w850] -> w838
              tunnel: w837 -> [w843 w849]
              tunnel: w829 -> [_ w848]
              tunnel: w827 -> [_ w847]
              tunnel: w801 -> [_ w846]
              tunnel: w817 -> [_ w845]
              tunnel: "Минуты 2" -> [_ w844]
              frame False {
              }
              frame True {
                n245 = case shown="True" w848 {
                  tunnel: [w873 w879] -> w852
                  tunnel: w849 -> [w872 w878]
                  tunnel: w846 -> [_ w877]
                  tunnel: w845 -> [_ w876]
                  tunnel: w844 -> [_ w875]
                  frame False {
                    n246 = Add(x=0, y=w872) -> (x+y=w873:i32)
                    n247 = Wait (ms)(milliseconds to wait=u32 500) -> ()  [unwired: 1 out]
                  }
                  frame True {
                    n248 = Type Cast(type="", x=w875) -> (*(type *) &x=w882:string)
                    n249 = Add(x=w875, y=w878) -> (x+y=w879:i32)
                    n250 = String Subset(string=w882, offset (0)=1, length (rest)=3 ("length (rest)")) -> (substring=w881:string)
                    n251 = Concatenate Strings("$2MJ\u0004+" ("write buffer"), w881) -> (w885:string)
                    n252 = VISA Write(VISA resource name=w876, write buffer=w885, error in (no error)=w877) -> ()  [unwired: 3 out]
                  }
                }
                n253 = case shown="True" w847 {
                  tunnel: [w855 w861] -> w850
                  tunnel: w851 -> [w854 w860]
                  tunnel: w845 -> [_ w863]
                  tunnel: w846 -> [_ w862]
                  tunnel: w844 -> [_ w857]
                  frame False {
                    n254 = Add(x=0, y=w854) -> (x+y=w855:i32)
                    n255 = Wait (ms)(milliseconds to wait=u32 500) -> ()  [unwired: 1 out]
                  }
                  frame True {
                    n256 = Multiply(x=w857, y=-1) -> (x*y=w859:i32)
                    n257 = Type Cast(type="", x=w859) -> (*(type *) &x=w866:string)
                    n258 = Add(x=w860, y=w857) -> (x+y=w861:i32)
                    n259 = String Subset(string=w866, offset (0)=1, length (rest)=3 ("length (rest)")) -> (substring=w865:string)
                    n260 = Concatenate Strings("$2MJ\u0004-" ("write buffer"), w865) -> (w869:string)
                    n261 = VISA Write(VISA resource name=w863, write buffer=w869, error in (no error)=w862) -> ()  [unwired: 3 out]
                  }
                }
              }
            }
            n262 = case shown="True" w822 {
              tunnel: [w903 w910] -> w834
              tunnel: w836 -> [w902 w905]
              tunnel: w817 -> [_ w906]
              tunnel: w801 -> [_ w907]
              frame False {
                n263 = Add(x=0, y=w902) -> (x+y=w903:i32)
                n264 = Wait (ms)(milliseconds to wait=u32 500) -> ()  [unwired: 1 out]
              }
              frame True {
                n265 = VISA Write(VISA resource name=w906, write buffer="$2MJ\u0004+\u0000\u0000<", error in (no error)=w907) -> ()  [unwired: 3 out]
                n266 = Add(x=60, y=w905) -> (x+y=w910:i32)
              }
            }
            n267 = case shown="True" w819 {
              tunnel: [w893 w896] -> w833
              tunnel: w835 -> [w892 w895]
              tunnel: w817 -> [_ w899]
              tunnel: w801 -> [_ w898]
              frame False {
                n268 = Add(x=0, y=w892) -> (x+y=w893:i32)
                n269 = Wait (ms)(milliseconds to wait=u32 500) -> ()  [unwired: 1 out]
              }
              frame True {
                n270 = Subtract(x=w895, y=60 ("x")) -> (x-y=w896:i32)
                n271 = VISA Write(VISA resource name=w899, write buffer="$2MJ\u0004-\u0000\u0000<", error in (no error)=w898) -> ()  [unwired: 3 out]
              }
            }
            n272 = for {
              N: 1 -> [_]
              tunnel: [w841] -> w797 mode=indexing
              n273 = local read "2"() -> (w841:i32)
            }
            n274 = Index Array(array=w797, index=0) -> (element=w799:i32)
          }
          frame #2 {
            # "Нулевое положение"
            n275 = Add(x=w926, y=w927) -> (x+y=w935:i32)
            n276 = Add(x=w924, y=w925) -> (x+y=w939:i32)
            n277 = Add(x=w939, y=w935) -> (x+y=w920:i32)
            n278 = Add(x=w920, y=w911) -> (x+y=w919:i32)
            n279 = Not Equal?(x=w919, y=0 ("x")) -> (x != y?=w932:bool)
            n280 = And(x=w932, y=w934) -> (x .and. y?=w941:bool)
            n281 = case shown="True" w941 {
              tunnel: [w966 w988] -> w913
              tunnel: w924 -> [w970 w985]
              tunnel: [w970 w984] -> w942
              tunnel: [w969 w983] -> w940
              tunnel: w919 -> [w966 w977]
              tunnel: [w967 w979] -> w938
              tunnel: [w968 w976] -> w931
              tunnel: w925 -> [w969 w975]
              tunnel: w930 -> [_ w974]
              tunnel: w929 -> [_ w973]
              tunnel: w926 -> [w968 w972]
              tunnel: w927 -> [w967 w971]
              frame False {
              }
              frame True {
                n282 = Greater?(x=w977, y=0) -> (0:w978:bool)
                n283 = Multiply(x=w971, y=0) -> (x*y=w979:i32)
                n284 = Multiply(x=w975, y=0) -> (x*y=w983:i32)
                n285 = case shown="True" w978 {
                  tunnel: w977 -> [w993 w1006]
                  tunnel: [0 0] -> w988
                  tunnel: w973 -> [w990 w1003]
                  tunnel: w974 -> [w989 w1002]
                  frame False {
                    n286 = Multiply(x=w993, y=-1) -> (x*y=w991:i32)
                    n287 = Type Cast(type="", x=w991) -> (*(type *) &x=w997:string)
                    n288 = String Subset(string=w997, offset (0)=1, length (rest)=3 ("length (rest)")) -> (substring=w996:string)
                    n289 = Concatenate Strings("$2MJ\u0004+" ("write buffer"), w996) -> (w1000:string)
                    n290 = VISA Write(VISA resource name=w990, write buffer=w1000, error in (no error)=w989) -> ()  [unwired: 3 out]
                  }
                  frame True {
                    n291 = Type Cast(type="", x=w1006) -> (*(type *) &x=w1009:string)
                    n292 = String Subset(string=w1009, offset (0)=1, length (rest)=3 ("length (rest)")) -> (substring=w1008:string)
                    n293 = Concatenate Strings("$2MJ\u0004-" ("write buffer"), w1008) -> (w1004:string)
                    n294 = VISA Write(VISA resource name=w1003, write buffer=w1004, error in (no error)=w1002) -> ()  [unwired: 3 out]
                  }
                }
                n295 = Multiply(x=w972, y=0) -> (x*y=w976:i32)
                n296 = Multiply(x=w985, y=0) -> (x*y=w984:i32)
              }
            }
            "положение в мин 2" <- w913
            n297 = Greater?(x=w913, y=0) -> (0:w937:bool)
            n298 = Number To Decimal String(number=w913, width (-)=i16 1) -> (decimal integer string=w922:string)
            n299 = case shown="False" w937 {
              tunnel: w913 -> [w949 w965]
              tunnel: [w953 w959] -> w917
              tunnel: [w943 w957] -> w916
              frame False {
                n300 = Multiply(x=-1, y=w949) -> (x*y=w948:i32)
                n301 = Quotient & Remainder(x=w948, y=60) -> (x-y*floor(x/y)=w952:i32, floor(x/y)=w944:i32)
                n302 = Multiply(x=-1, y=w944) -> (x*y=w943:i32)
                n303 = Number To Decimal String(number=w944) -> (decimal integer string=w950:string)  [unwired: 1 in]
                n304 = Number To Decimal String(number=w952) -> (decimal integer string=w951:string)  [unwired: 1 in]
                n305 = Concatenate Strings("-" ("string"), w950, "°" ("string"), w951, "'" ("string")) -> (w953:string)
              }
              frame True {
                n306 = Quotient & Remainder(x=w965, y=60) -> (x-y*floor(x/y)=w958:i32, floor(x/y)=w957:i32)
                n307 = Number To Decimal String(number=w958) -> (decimal integer string=w960:string)  [unwired: 1 in]
                n308 = Number To Decimal String(number=w957) -> (decimal integer string=w961:string)  [unwired: 1 in]
                n309 = Concatenate Strings(w961, "°" ("string"), w960, "'" ("string")) -> (w959:string)
              }
            }
            "положение шд 2" <- w916
            "текущее положение 2" <- w917
            n310 = Concatenate Strings(w922, "'" ("string")) -> (→"положение в минутах 2":string)
            n311 = Format Into String(w913) -> (resulting string=w914:string)  [unwired: 3 in, 1 out]
            n312 = call <vilib>:"Space Constant.vi"() -> ("String"=w912:string)
            n313 = Concatenate Strings(w912, w914) -> (→"text2":string)
          }
          frame #3 {
            # "Задача нуля"
            n314 = case shown="True" w1013 {
              tunnel: [w1025 w1036] -> w1021
              tunnel: w1020 -> [w1025 w1037]
              tunnel: w1019 -> [w1024 w1033]
              tunnel: [w1024 w1032] -> w1018
              tunnel: [w1023 w1029] -> w1017
              tunnel: [w1022 w1028] -> w1016
              tunnel: w1015 -> [w1023 w1027]
              tunnel: w1014 -> [w1022 w1026]
              frame False {
              }
              frame True {
                n315 = Multiply(x=w1033, y=0) -> (x*y=w1032:i32)
                n316 = Multiply(x=w1037, y=0) -> (x*y=w1036:i32)
                n317 = Multiply(x=w1026, y=0) -> (x*y=w1028:i32)
                n318 = Multiply(x=w1027, y=0) -> (x*y=w1029:i32)
              }
            }
          }
        }
        n319 = flat-sequence {
          tunnel: w100 -> [w248]
          tunnel: w101 -> [w249]
          tunnel: [w249] -> w122
          tunnel: [w248] -> w121
          tunnel: ["Вращение по градусам +  4"] -> w120
          tunnel: ["Вращение по градусам -  4"] -> w119
          tunnel: ["Вернуться в нулевое положение 4"] -> w118
          tunnel: ["Задать текущее положение нулевым 4"] -> w117
          tunnel: ["Установка минут 4"] -> w116
          tunnel: w122 -> [w273]
          tunnel: w121 -> [w257]
          tunnel: [w296] -> w115
          tunnel: w98 -> [w293]
          tunnel: w96 -> [w295]
          tunnel: [w294] -> w114
          tunnel: w94 -> [w292]
          tunnel: w92 -> [w291]
          tunnel: w120 -> [w277]
          tunnel: w119 -> [w276]
          tunnel: [w290] -> w113
          tunnel: [w289] -> w112
          tunnel: [w274] -> w111
          tunnel: w118 -> [w274]
          tunnel: [w257] -> w110
          tunnel: [w273] -> w109
          tunnel: [w272] -> w108
          tunnel: w117 -> [w272]
          tunnel: w116 -> [w266]
          tunnel: [w255] -> w107
          tunnel: w115 -> [w380]
          tunnel: w114 -> [w381]
          tunnel: [w398] -> w106
          tunnel: [w396] -> w105
          tunnel: w113 -> [w382]
          tunnel: w112 -> [w383]
          tunnel: [w387] -> w104
          tunnel: [w394] -> w103
          tunnel: w111 -> [w390]
          tunnel: w110 -> [w386]
          tunnel: w109 -> [w385]
          tunnel: w108 -> [w384]
          tunnel: [w384] -> w102
          tunnel: w107 -> [w370]
          tunnel: [w477] -> w97
          tunnel: [w474] -> w95
          tunnel: w106 -> [w476]
          tunnel: w105 -> [w475]
          tunnel: [w473] -> w93
          tunnel: [w472] -> w91
          tunnel: w104 -> [w471]
          tunnel: w103 -> [w470]
          tunnel: w102 -> [w469]
          frame #0 {
            n320 = Wait Until Next ms Multiple(millisecond multiple=u32 300) -> ()  [unwired: 1 out]
          }
          frame #1 {
            # "Остановка двигателя"
            n321 = Greater?(x="Минуты 4", y=0) -> (0:w264:bool)
            n322 = case shown="True" "Stop двигатель 4" {
              tunnel: w273 -> [_ w344]
              tunnel: w257 -> [_ w343]
              frame False {
              }
              frame True {
                n323 = Wait (ms)(milliseconds to wait=u32 500) -> ()  [unwired: 1 out]
                n324 = VISA Write(VISA resource name=w344, write buffer="$4MS\u0001", error in (no error)=w343) -> ()  [unwired: 3 out]
              }
            }
            n325 = Not Equal?(x="Минуты 4", y=0) -> (x != y?=w263:bool)
            n326 = local read "положение в мин 4"() -> (w256:i32)
            n327 = Add(x="Минуты 4", y=w256) -> (x+y=w287:i32)
            n328 = Add(x="Минуты 4", y=w256) -> (x+y=w259:i32)
            n329 = Not Equal?(x="Минуты 4", y=0) -> (x != y?=w261:bool)
            n330 = Add(x=w256, y=60) -> (x+y=w282:i32)
            n331 = Subtract(x=w256, y=60) -> (x-y=w269:i32)
            n332 = Not(x=w264) -> (.not. x?=w265:bool)
            n333 = Greater Or Equal?(x=w259, y=-600) -> (x >= y?=w260:bool)
            n334 = Less Or Equal?(x=w287, y=11400) -> (x <= y?=w262:bool)
            n335 = Less Or Equal?(x=w282, y=11390) -> (x <= y?=w279:bool)
            n336 = Greater Or Equal?(x=w269, y=-590) -> (x >= y?=w270:bool)
            n337 = Compound Arithmetic op=AND(w265, w261, w260) -> (w283:bool)
            n338 = And(x=w277, y=w279) -> (x .and. y?=w278:bool)
            n339 = And(x=w276, y=w270) -> (x .and. y?=w275:bool)
            n340 = Compound Arithmetic op=AND(w264, w263, w262) -> (w285:bool)
            n341 = case shown="True" w266 {
              tunnel: [w299 w308] -> w296
              tunnel: w295 -> [w298 w307]
              tunnel: [w298 w306] -> w294
              tunnel: w293 -> [w299 w305]
              tunnel: w285 -> [_ w304]
              tunnel: w283 -> [_ w303]
              tunnel: w257 -> [_ w302]
              tunnel: w273 -> [_ w301]
              tunnel: "Минуты 4" -> [_ w300]
              frame False {
              }
              frame True {
                n342 = case shown="True" w304 {
                  tunnel: [w329 w335] -> w308
                  tunnel: w305 -> [w328 w334]
                  tunnel: w302 -> [_ w333]
                  tunnel: w301 -> [_ w332]
                  tunnel: w300 -> [_ w331]
                  frame False {
                    n343 = Add(x=0, y=w328) -> (x+y=w329:i32)
                    n344 = Wait (ms)(milliseconds to wait=u32 500) -> ()  [unwired: 1 out]
                  }
                  frame True {
                    n345 = Type Cast(type="", x=w331) -> (*(type *) &x=w338:string)
                    n346 = Add(x=w331, y=w334) -> (x+y=w335:i32)
                    n347 = String Subset(string=w338, offset (0)=1, length (rest)=3 ("length (rest)")) -> (substring=w337:string)
                    n348 = Concatenate Strings("$4MJ\u0004+" ("write buffer"), w337) -> (w341:string)
                    n349 = VISA Write(VISA resource name=w332, write buffer=w341, error in (no error)=w333) -> ()  [unwired: 3 out]
                  }
                }
                n350 = case shown="True" w303 {
                  tunnel: [w311 w317] -> w306
                  tunnel: w307 -> [w310 w316]
                  tunnel: w301 -> [_ w319]
                  tunnel: w302 -> [_ w318]
                  tunnel: w300 -> [_ w313]
                  frame False {
                    n351 = Add(x=0, y=w310) -> (x+y=w311:i32)
                    n352 = Wait (ms)(milliseconds to wait=u32 500) -> ()  [unwired: 1 out]
                  }
                  frame True {
                    n353 = Multiply(x=w313, y=-1) -> (x*y=w315:i32)
                    n354 = Type Cast(type="", x=w315) -> (*(type *) &x=w322:string)
                    n355 = Add(x=w316, y=w313) -> (x+y=w317:i32)
                    n356 = String Subset(string=w322, offset (0)=1, length (rest)=3 ("length (rest)")) -> (substring=w321:string)
                    n357 = Concatenate Strings("$4MJ\u0004-" ("write buffer"), w321) -> (w325:string)
                    n358 = VISA Write(VISA resource name=w319, write buffer=w325, error in (no error)=w318) -> ()  [unwired: 3 out]
                  }
                }
              }
            }
            n359 = case shown="True" w278 {
              tunnel: [w359 w366] -> w290
              tunnel: w292 -> [w358 w361]
              tunnel: w273 -> [_ w362]
              tunnel: w257 -> [_ w363]
              frame False {
                n360 = Add(x=0, y=w358) -> (x+y=w359:i32)
                n361 = Wait (ms)(milliseconds to wait=u32 500) -> ()  [unwired: 1 out]
              }
              frame True {
                n362 = VISA Write(VISA resource name=w362, write buffer="$4MJ\u0004+\u0000\u0000<", error in (no error)=w363) -> ()  [unwired: 3 out]
                n363 = Add(x=60, y=w361) -> (x+y=w366:i32)
              }
            }
            n364 = case shown="True" w275 {
              tunnel: [w349 w352] -> w289
              tunnel: w291 -> [w348 w351]
              tunnel: w273 -> [_ w355]
              tunnel: w257 -> [_ w354]
              frame False {
                n365 = Add(x=0, y=w348) -> (x+y=w349:i32)
                n366 = Wait (ms)(milliseconds to wait=u32 500) -> ()  [unwired: 1 out]
              }
              frame True {
                n367 = Subtract(x=w351, y=60 ("x")) -> (x-y=w352:i32)
                n368 = VISA Write(VISA resource name=w355, write buffer="$4MJ\u0004-\u0000\u0000<", error in (no error)=w354) -> ()  [unwired: 3 out]
              }
            }
            n369 = for {
              N: 1 -> [_]
              tunnel: [w297] -> w253 mode=indexing
              n370 = local read "4"() -> (w297:i32)
            }
            n371 = Index Array(array=w253, index=0) -> (element=w255:i32)
          }
          frame #2 {
            # "Нулевое положение"
            n372 = Add(x=w382, y=w383) -> (x+y=w391:i32)
            n373 = Add(x=w380, y=w381) -> (x+y=w395:i32)
            n374 = Add(x=w395, y=w391) -> (x+y=w376:i32)
            n375 = Add(x=w376, y=w370) -> (x+y=w375:i32)
            n376 = Not Equal?(x=w375, y=0 ("x")) -> (x != y?=w388:bool)
            n377 = And(x=w388, y=w390) -> (x .and. y?=w397:bool)
            n378 = case shown="True" w397 {
              tunnel: [w422 w444] -> w372
              tunnel: w380 -> [w426 w441]
              tunnel: [w426 w440] -> w398
              tunnel: [w425 w439] -> w396
              tunnel: w375 -> [w422 w433]
              tunnel: [w423 w435] -> w394
              tunnel: [w424 w432] -> w387
              tunnel: w381 -> [w425 w431]
              tunnel: w386 -> [_ w430]
              tunnel: w385 -> [_ w429]
              tunnel: w382 -> [w424 w428]
              tunnel: w383 -> [w423 w427]
              frame False {
              }
              frame True {
                n379 = Greater?(x=w433, y=0) -> (0:w434:bool)
                n380 = Multiply(x=w427, y=0) -> (x*y=w435:i32)
                n381 = Multiply(x=w431, y=0) -> (x*y=w439:i32)
                n382 = case shown="True" w434 {
                  tunnel: w433 -> [w449 w462]
                  tunnel: [0 0] -> w444
                  tunnel: w429 -> [w446 w459]
                  tunnel: w430 -> [w445 w458]
                  frame False {
                    n383 = Multiply(x=w449, y=-1) -> (x*y=w447:i32)
                    n384 = Type Cast(type="", x=w447) -> (*(type *) &x=w453:string)
                    n385 = String Subset(string=w453, offset (0)=1, length (rest)=3 ("length (rest)")) -> (substring=w452:string)
                    n386 = Concatenate Strings("$4MJ\u0004+" ("write buffer"), w452) -> (w456:string)
                    n387 = VISA Write(VISA resource name=w446, write buffer=w456, error in (no error)=w445) -> ()  [unwired: 3 out]
                  }
                  frame True {
                    n388 = Type Cast(type="", x=w462) -> (*(type *) &x=w465:string)
                    n389 = String Subset(string=w465, offset (0)=1, length (rest)=3 ("length (rest)")) -> (substring=w464:string)
                    n390 = Concatenate Strings("$4MJ\u0004-" ("write buffer"), w464) -> (w460:string)
                    n391 = VISA Write(VISA resource name=w459, write buffer=w460, error in (no error)=w458) -> ()  [unwired: 3 out]
                  }
                }
                n392 = Multiply(x=w428, y=0) -> (x*y=w432:i32)
                n393 = Multiply(x=w441, y=0) -> (x*y=w440:i32)
              }
            }
            "положение в мин 4" <- w372
            n394 = Greater?(x=w372, y=0) -> (0:w393:bool)
            n395 = Number To Decimal String(number=w372, width (-)=i16 1) -> (decimal integer string=w378:string)
            n396 = case shown="False" w393 {
              tunnel: w372 -> [w405 w421]
              tunnel: [w409 w415] -> w368
              tunnel: [w399 w413] -> w369
              frame False {
                n397 = Multiply(x=-1, y=w405) -> (x*y=w404:i32)
                n398 = Quotient & Remainder(x=w404, y=60) -> (x-y*floor(x/y)=w408:i32, floor(x/y)=w400:i32)
                n399 = Multiply(x=-1, y=w400) -> (x*y=w399:i32)
                n400 = Number To Decimal String(number=w400) -> (decimal integer string=w406:string)  [unwired: 1 in]
                n401 = Number To Decimal String(number=w408) -> (decimal integer string=w407:string)  [unwired: 1 in]
                n402 = Concatenate Strings("-" ("string"), w406, "°" ("string"), w407, "'" ("string")) -> (w409:string)
              }
              frame True {
                n403 = Quotient & Remainder(x=w421, y=60) -> (x-y*floor(x/y)=w414:i32, floor(x/y)=w413:i32)
                n404 = Number To Decimal String(number=w414) -> (decimal integer string=w416:string)  [unwired: 1 in]
                n405 = Number To Decimal String(number=w413) -> (decimal integer string=w417:string)  [unwired: 1 in]
                n406 = Concatenate Strings(w417, "°" ("string"), w416, "'" ("string")) -> (w415:string)
              }
            }
            "положение шд 4" <- w369
            "текущее положение 4" <- w368
            n407 = Concatenate Strings(w378, "'" ("string")) -> (→"положение в минутах 4":string)
            n408 = Format Into String(w372) -> (resulting string=w373:string)  [unwired: 3 in, 1 out]
            n409 = call <vilib>:"Space Constant.vi"() -> ("String"=w371:string)
            n410 = Concatenate Strings(w371, w373) -> (→"text4":string)
          }
          frame #3 {
            # "Задача нуля"
            n411 = case shown="True" w469 {
              tunnel: [w481 w492] -> w477
              tunnel: w476 -> [w481 w493]
              tunnel: w475 -> [w480 w489]
              tunnel: [w480 w488] -> w474
              tunnel: [w479 w485] -> w473
              tunnel: [w478 w484] -> w472
              tunnel: w471 -> [w479 w483]
              tunnel: w470 -> [w478 w482]
              frame False {
              }
              frame True {
                n412 = Multiply(x=w489, y=0) -> (x*y=w488:i32)
                n413 = Multiply(x=w493, y=0) -> (x*y=w492:i32)
                n414 = Multiply(x=w482, y=0) -> (x*y=w484:i32)
                n415 = Multiply(x=w483, y=0) -> (x*y=w485:i32)
              }
            }
          }
        }
        n416 = case shown="True" "Блокировать трубку №2" {
          frame False {
            n417 = property on="Stop двигатель 2" class="Bool"("DisabledEnum"=T3."Enabled" ("Disabled")) -> ()  [unwired: 2 in, 2 out]
            n418 = property on="Вернуться в нулевое положение 2" class="Bool"("DisabledEnum"=T3."Enabled" ("Disabled")) -> ()  [unwired: 2 in, 2 out]
            n419 = property on="Вращение по градусам +  2" class="Bool"("DisabledEnum"=T3."Enabled" ("Disabled")) -> ()  [unwired: 2 in, 2 out]
            n420 = property on="текущее положение 2" class="Str"("DisabledEnum"=T3."Enabled" ("Disabled")) -> ()  [unwired: 2 in, 2 out]
            n421 = property on="Установка минут 2" class="Bool"("DisabledEnum"=T3."Enabled" ("Disabled")) -> ()  [unwired: 2 in, 2 out]
            n422 = property on="Вращение по градусам -  2" class="Bool"("DisabledEnum"=T3."Enabled" ("Disabled")) -> ()  [unwired: 2 in, 2 out]
            n423 = property on="Задать текущее положение нулевым 2" class="Bool"("DisabledEnum"=T3."Enabled" ("Disabled")) -> ()  [unwired: 2 in, 2 out]
            n424 = property on="Минуты 2" class="DigNum (strict)"("DisabledEnum"=T3."Enabled" ("Disabled")) -> ()  [unwired: 2 in, 2 out]
            n425 = property on="положение шд 2" class="Knob (strict)"("DisabledEnum"=T3."Enabled" ("Disabled")) -> ()  [unwired: 2 in, 2 out]
            n426 = property on="положение в минутах 2" class="Str"("DisabledEnum"=T3."Enabled" ("Disabled")) -> ()  [unwired: 2 in, 2 out]
          }
          frame True {
            n427 = property on="Вернуться в нулевое положение 2" class="Bool"("DisabledEnum"=T3."Disabled and Grayed Out" ("Disabled")) -> ()  [unwired: 2 in, 2 out]
            n428 = property on="положение шд 2" class="Knob (strict)"("DisabledEnum"=T3."Disabled and Grayed Out" ("Disabled")) -> ()  [unwired: 2 in, 2 out]
            n429 = property on="текущее положение 2" class="Str"("DisabledEnum"=T3."Disabled and Grayed Out" ("Disabled")) -> ()  [unwired: 2 in, 2 out]
            n430 = property on="Stop двигатель 2" class="Bool"("DisabledEnum"=T3."Disabled and Grayed Out" ("Disabled")) -> ()  [unwired: 2 in, 2 out]
            n431 = property on="Вращение по градусам +  2" class="Bool"("DisabledEnum"=T3."Disabled and Grayed Out" ("Disabled")) -> ()  [unwired: 2 in, 2 out]
            n432 = property on="Вращение по градусам -  2" class="Bool"("DisabledEnum"=T3."Disabled and Grayed Out" ("Disabled")) -> ()  [unwired: 2 in, 2 out]
            n433 = property on="Задать текущее положение нулевым 2" class="Bool"("DisabledEnum"=T3."Disabled and Grayed Out" ("Disabled")) -> ()  [unwired: 2 in, 2 out]
            n434 = property on="Минуты 2" class="DigNum (strict)"("DisabledEnum"=T3."Disabled and Grayed Out" ("Disabled")) -> ()  [unwired: 2 in, 2 out]
            n435 = property on="Установка минут 2" class="Bool"("DisabledEnum"=T3."Disabled and Grayed Out" ("Disabled")) -> ()  [unwired: 2 in, 2 out]
            n436 = property on="положение в минутах 2" class="Str"("DisabledEnum"=T3."Disabled and Grayed Out" ("Disabled")) -> ()  [unwired: 2 in, 2 out]
          }
        }
        n437 = case shown="False" "Блокировать стол №3" {
          frame False {
            n438 = property on="Stop двигатель 3" class="Bool"("DisabledEnum"=T3."Enabled" ("Disabled")) -> ()  [unwired: 2 in, 2 out]
            n439 = property on="Вернуться в нулевое положение 3" class="Bool"("DisabledEnum"=T3."Enabled" ("Disabled")) -> ()  [unwired: 2 in, 2 out]
            n440 = property on="Вращение по градусам +  3" class="Bool"("DisabledEnum"=T3."Enabled" ("Disabled")) -> ()  [unwired: 2 in, 2 out]
            n441 = property on="текущее положение 3" class="Str"("DisabledEnum"=T3."Enabled" ("Disabled")) -> ()  [unwired: 2 in, 2 out]
            n442 = property on="Установка минут 3" class="Bool"("DisabledEnum"=T3."Enabled" ("Disabled")) -> ()  [unwired: 2 in, 2 out]
            n443 = property on="Вращение по градусам -  3" class="Bool"("DisabledEnum"=T3."Enabled" ("Disabled")) -> ()  [unwired: 2 in, 2 out]
            n444 = property on="Задать текущее положение нулевым 3" class="Bool"("DisabledEnum"=T3."Enabled" ("Disabled")) -> ()  [unwired: 2 in, 2 out]
            n445 = property on="Минуты 3" class="DigNum (strict)"("DisabledEnum"=T3."Enabled" ("Disabled")) -> ()  [unwired: 2 in, 2 out]
            n446 = property on="положение шд 3" class="Knob (strict)"("DisabledEnum"=T3."Enabled" ("Disabled")) -> ()  [unwired: 2 in, 2 out]
            n447 = property on="положение в минутах 3" class="Str"("DisabledEnum"=T3."Enabled" ("Disabled")) -> ()  [unwired: 2 in, 2 out]
          }
          frame True {
            n448 = property on="Вернуться в нулевое положение 3" class="Bool"("DisabledEnum"=T3."Disabled and Grayed Out" ("Disabled")) -> ()  [unwired: 2 in, 2 out]
            n449 = property on="положение шд 3" class="Knob (strict)"("DisabledEnum"=T3."Disabled and Grayed Out" ("Disabled")) -> ()  [unwired: 2 in, 2 out]
            n450 = property on="текущее положение 3" class="Str"("DisabledEnum"=T3."Disabled and Grayed Out" ("Disabled")) -> ()  [unwired: 2 in, 2 out]
            n451 = property on="Stop двигатель 3" class="Bool"("DisabledEnum"=T3."Disabled and Grayed Out" ("Disabled")) -> ()  [unwired: 2 in, 2 out]
            n452 = property on="Вращение по градусам +  3" class="Bool"("DisabledEnum"=T3."Disabled and Grayed Out" ("Disabled")) -> ()  [unwired: 2 in, 2 out]
            n453 = property on="Вращение по градусам -  3" class="Bool"("DisabledEnum"=T3."Disabled and Grayed Out" ("Disabled")) -> ()  [unwired: 2 in, 2 out]
            n454 = property on="Задать текущее положение нулевым 3" class="Bool"("DisabledEnum"=T3."Disabled and Grayed Out" ("Disabled")) -> ()  [unwired: 2 in, 2 out]
            n455 = property on="Минуты 3" class="DigNum (strict)"("DisabledEnum"=T3."Disabled and Grayed Out" ("Disabled")) -> ()  [unwired: 2 in, 2 out]
            n456 = property on="Установка минут 3" class="Bool"("DisabledEnum"=T3."Disabled and Grayed Out" ("Disabled")) -> ()  [unwired: 2 in, 2 out]
            n457 = property on="положение в минутах 3" class="Str"("DisabledEnum"=T3."Disabled and Grayed Out" ("Disabled")) -> ()  [unwired: 2 in, 2 out]
          }
        }
        n458 = case shown="False" "Блокировать зеркало №1" {
          frame False {
            n459 = property on="Stop двигатель" class="Bool"("DisabledEnum"=T3."Enabled" ("Disabled")) -> ()  [unwired: 2 in, 2 out]
            n460 = property on="Вернуться в нулевое положение" class="Bool"("DisabledEnum"=T3."Enabled" ("Disabled")) -> ()  [unwired: 2 in, 2 out]
            n461 = property on="Вращение по градусам +" class="Bool"("DisabledEnum"=T3."Enabled" ("Disabled")) -> ()  [unwired: 2 in, 2 out]
            n462 = property on="текущее положение" class="Str"("DisabledEnum"=T3."Enabled" ("Disabled")) -> ()  [unwired: 2 in, 2 out]
            n463 = property on="Установка минут" class="Bool"("DisabledEnum"=T3."Enabled" ("Disabled")) -> ()  [unwired: 2 in, 2 out]
            n464 = property on="Вращение по градусам -" class="Bool"("DisabledEnum"=T3."Enabled" ("Disabled")) -> ()  [unwired: 2 in, 2 out]
            n465 = property on="Задать текущее положение нулевым" class="Bool"("DisabledEnum"=T3."Enabled" ("Disabled")) -> ()  [unwired: 2 in, 2 out]
            n466 = property on="Минуты" class="DigNum (strict)"("DisabledEnum"=T3."Enabled" ("Disabled")) -> ()  [unwired: 2 in, 2 out]
            n467 = property on="положение шд" class="Knob (strict)"("DisabledEnum"=T3."Enabled" ("Disabled")) -> ()  [unwired: 2 in, 2 out]
            n468 = property on="положение в минутах 1" class="Str"("DisabledEnum"=T3."Enabled" ("Disabled")) -> ()  [unwired: 2 in, 2 out]
          }
          frame True {
            n469 = property on="Вернуться в нулевое положение" class="Bool"("DisabledEnum"=T3."Disabled and Grayed Out" ("Disabled")) -> ()  [unwired: 2 in, 2 out]
            n470 = property on="положение шд" class="Knob (strict)"("DisabledEnum"=T3."Disabled and Grayed Out" ("Disabled")) -> ()  [unwired: 2 in, 2 out]
            n471 = property on="текущее положение" class="Str"("DisabledEnum"=T3."Disabled and Grayed Out" ("Disabled")) -> ()  [unwired: 2 in, 2 out]
            n472 = property on="Stop двигатель" class="Bool"("DisabledEnum"=T3."Disabled and Grayed Out" ("Disabled")) -> ()  [unwired: 2 in, 2 out]
            n473 = property on="Вращение по градусам +" class="Bool"("DisabledEnum"=T3."Disabled and Grayed Out" ("Disabled")) -> ()  [unwired: 2 in, 2 out]
            n474 = property on="Вращение по градусам -" class="Bool"("DisabledEnum"=T3."Disabled and Grayed Out" ("Disabled")) -> ()  [unwired: 2 in, 2 out]
            n475 = property on="Задать текущее положение нулевым" class="Bool"("DisabledEnum"=T3."Disabled and Grayed Out" ("Disabled")) -> ()  [unwired: 2 in, 2 out]
            n476 = property on="Минуты" class="DigNum (strict)"("DisabledEnum"=T3."Disabled and Grayed Out" ("Disabled")) -> ()  [unwired: 2 in, 2 out]
            n477 = property on="Установка минут" class="Bool"("DisabledEnum"=T3."Disabled and Grayed Out" ("Disabled")) -> ()  [unwired: 2 in, 2 out]
            n478 = property on="положение в минутах 1" class="Str"("DisabledEnum"=T3."Disabled and Grayed Out" ("Disabled")) -> ()  [unwired: 2 in, 2 out]
          }
        }
        n479 = case shown="False" "Блокировать стол №3 2" {
          frame False {
            n480 = property on="Stop двигатель 4" class="Bool"("DisabledEnum"=T3."Enabled" ("Disabled")) -> ()  [unwired: 2 in, 2 out]
            n481 = property on="Вернуться в нулевое положение 4" class="Bool"("DisabledEnum"=T3."Enabled" ("Disabled")) -> ()  [unwired: 2 in, 2 out]
            n482 = property on="Вращение по градусам +  4" class="Bool"("DisabledEnum"=T3."Enabled" ("Disabled")) -> ()  [unwired: 2 in, 2 out]
            n483 = property on="текущее положение 4" class="Str"("DisabledEnum"=T3."Enabled" ("Disabled")) -> ()  [unwired: 2 in, 2 out]
            n484 = property on="Установка минут 4" class="Bool"("DisabledEnum"=T3."Enabled" ("Disabled")) -> ()  [unwired: 2 in, 2 out]
            n485 = property on="Вращение по градусам -  4" class="Bool"("DisabledEnum"=T3."Enabled" ("Disabled")) -> ()  [unwired: 2 in, 2 out]
            n486 = property on="Задать текущее положение нулевым 4" class="Bool"("DisabledEnum"=T3."Enabled" ("Disabled")) -> ()  [unwired: 2 in, 2 out]
            n487 = property on="Минуты 4" class="DigNum (strict)"("DisabledEnum"=T3."Enabled" ("Disabled")) -> ()  [unwired: 2 in, 2 out]
            n488 = property on="положение шд 4" class="Knob (strict)"("DisabledEnum"=T3."Enabled" ("Disabled")) -> ()  [unwired: 2 in, 2 out]
            n489 = property on="положение в минутах 4" class="Str"("DisabledEnum"=T3."Enabled" ("Disabled")) -> ()  [unwired: 2 in, 2 out]
          }
          frame True {
            n490 = property on="Вернуться в нулевое положение 4" class="Bool"("DisabledEnum"=T3."Disabled and Grayed Out" ("Disabled")) -> ()  [unwired: 2 in, 2 out]
            n491 = property on="положение шд 4" class="Knob (strict)"("DisabledEnum"=T3."Disabled and Grayed Out" ("Disabled")) -> ()  [unwired: 2 in, 2 out]
            n492 = property on="текущее положение 4" class="Str"("DisabledEnum"=T3."Disabled and Grayed Out" ("Disabled")) -> ()  [unwired: 2 in, 2 out]
            n493 = property on="Stop двигатель 4" class="Bool"("DisabledEnum"=T3."Disabled and Grayed Out" ("Disabled")) -> ()  [unwired: 2 in, 2 out]
            n494 = property on="Вращение по градусам +  4" class="Bool"("DisabledEnum"=T3."Disabled and Grayed Out" ("Disabled")) -> ()  [unwired: 2 in, 2 out]
            n495 = property on="Вращение по градусам -  4" class="Bool"("DisabledEnum"=T3."Disabled and Grayed Out" ("Disabled")) -> ()  [unwired: 2 in, 2 out]
            n496 = property on="Задать текущее положение нулевым 4" class="Bool"("DisabledEnum"=T3."Disabled and Grayed Out" ("Disabled")) -> ()  [unwired: 2 in, 2 out]
            n497 = property on="Минуты 4" class="DigNum (strict)"("DisabledEnum"=T3."Disabled and Grayed Out" ("Disabled")) -> ()  [unwired: 2 in, 2 out]
            n498 = property on="Установка минут 4" class="Bool"("DisabledEnum"=T3."Disabled and Grayed Out" ("Disabled")) -> ()  [unwired: 2 in, 2 out]
            n499 = property on="положение в минутах 4" class="Str"("DisabledEnum"=T3."Disabled and Grayed Out" ("Disabled")) -> ()  [unwired: 2 in, 2 out]
          }
        }
      }
      n500 = Close File(refnum=w86) -> ()  [unwired: 1 in, 2 out]
    }
  }
